vi "TCP_Request Triage.vi"(10 "Message":string) -> (0 "Value":string, 1 "Variable":string, 3 "Request":string)   [LabVIEW 2019]
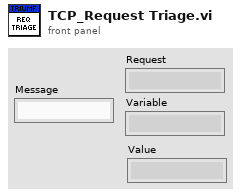
[diagram p1: front panel]
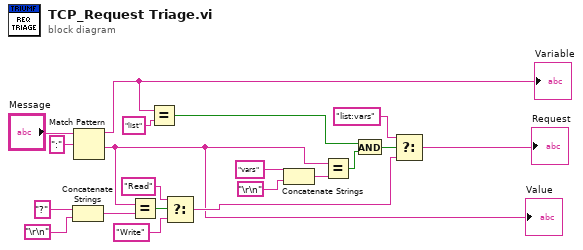
[diagram p0: block diagram]
diagram:
  n1 = Concatenate Strings("?" ("y"), "\r\n") -> (w8:string)
  n2 = Match Pattern(string="Message", regular expression=":") -> (before substring=w17:string, after substring=w18:string)  [unwired: 1 in, 2 out]
  "Variable" <- w17
  "Value" <- w18
  n3 = Equal?(x=w18, y=w8) -> (x = y?=w3:bool)
  n4 = Equal?(x=w17, y="list") -> (x = y?=w14:bool)
  n5 = Select(t="Read" ("y"), s=w3, f="Write" ("y")) -> (s? t:f=w20:string)
  n6 = Concatenate Strings("vars" ("y"), "\r\n") -> (w12:string)
  n7 = Equal?(x=w18, y=w12) -> (x = y?=w13:bool)
  n8 = And(x=w14, y=w13) -> (x .and. y?=w15:bool)
  n9 = Select(t="list:vars" ("y"), s=w15, f=w20) -> (s? t:f=→"Request":string)
